vi "TagBus_Read Table (DVR).vi"(10 "Index Array":i32[](array[numeric]), 11 "Data Value Reference in":refnum<data-value>) -> (2 "Value Array":dbl[](array[numeric]), 3 "Data Value Reference out":refnum<data-value>)   [LabVIEW 2015, in "TagBus.lvclass"]
uses:
  TagBus.lvclass
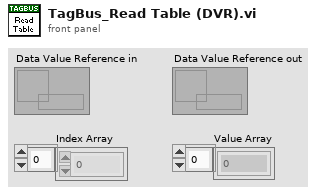
[diagram p1: front panel]
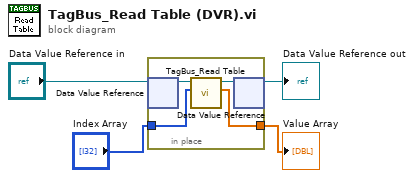
[diagram p0: block diagram]
diagram:
  n1 = in-place {
    in-place-border: [w8] -> w4
    in-place-border: "Index Array" -> [w5]
    n2 = in-place-dvr #1("Data Value Reference in") -> (w6:refnum<class "TagBus.lvclass">)  [unwired: 1 out]
    n3 = call "TagBus_Read Table.vi"("Index Array"=w5, "TagBus"=w6) -> ("Value Array"=w8:dbl[], "TagBus out"=w7:refnum<class "TagBus.lvclass">)  [unwired: 8 in]
    n4 = in-place-dvr #1(w7) -> (→"Data Value Reference out":refnum<data-value>)  [unwired: 1 out]
  }
  "Value Array" <- w4
